vi "autofocus-mainvi.vi"() -> ()   [LabVIEW 2014]
uses:
  Stage Control/Stage SubVis/move stage.ctl
  autofocus-globals.vi
  tirf-lock-globals.vi
  <vilib>/Analysis/polynomials.llb/1D Polynomial Evaluation (DBL).vi
  <vilib>/Analysis/NI_AALPro.lvlib
panel:
  in  "Close laser shutter when autofocus is done?":bool
  in  "Close camera shutter during autofocus?":bool
  out "delta Z":dbl format="%#_13g"
  out "Calibration curve and fit":cluster{"QPD position":dbl[], "z (um)":ext[]}[](graph)
  out "Power":dbl format="%#_13g"
  out "Error Out":errorcluster
  in  "Error In":errorcluster
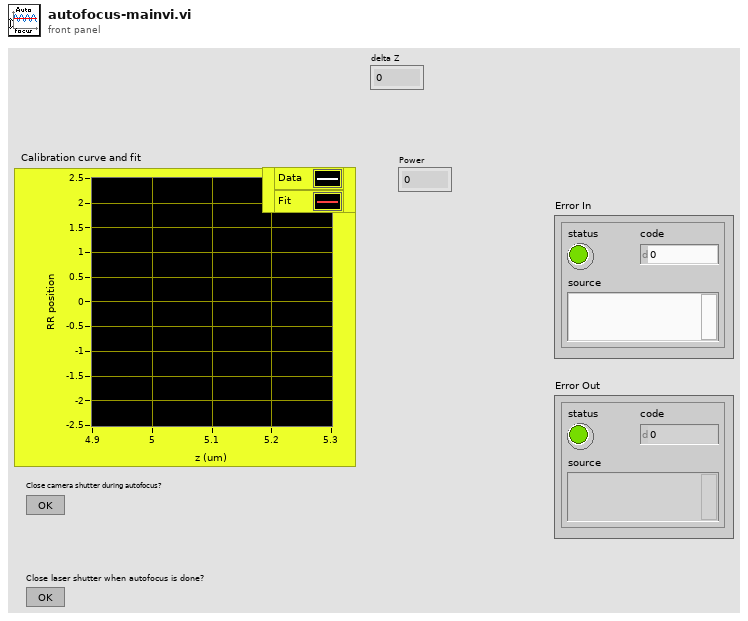
[diagram p1: front panel]
types:
  T1 = typedef "move stage.ctl" = cluster{"dx (um) (0 -> ignore)":ext, "dy (um) (0 -> ignore)":ext, "dz (um) (0 -> ignore)":ext, "Re-center x,y":bool, "Re-center z":bool, "x (um) (-1 -> ignore)":dbl, "y (um) (-1 -> ignore)":dbl, "z (um) (-1 -> ignore)":dbl}
  T2 = cluster{"QPD position":dbl[], "Best Polynomial Fit":dbl[]}
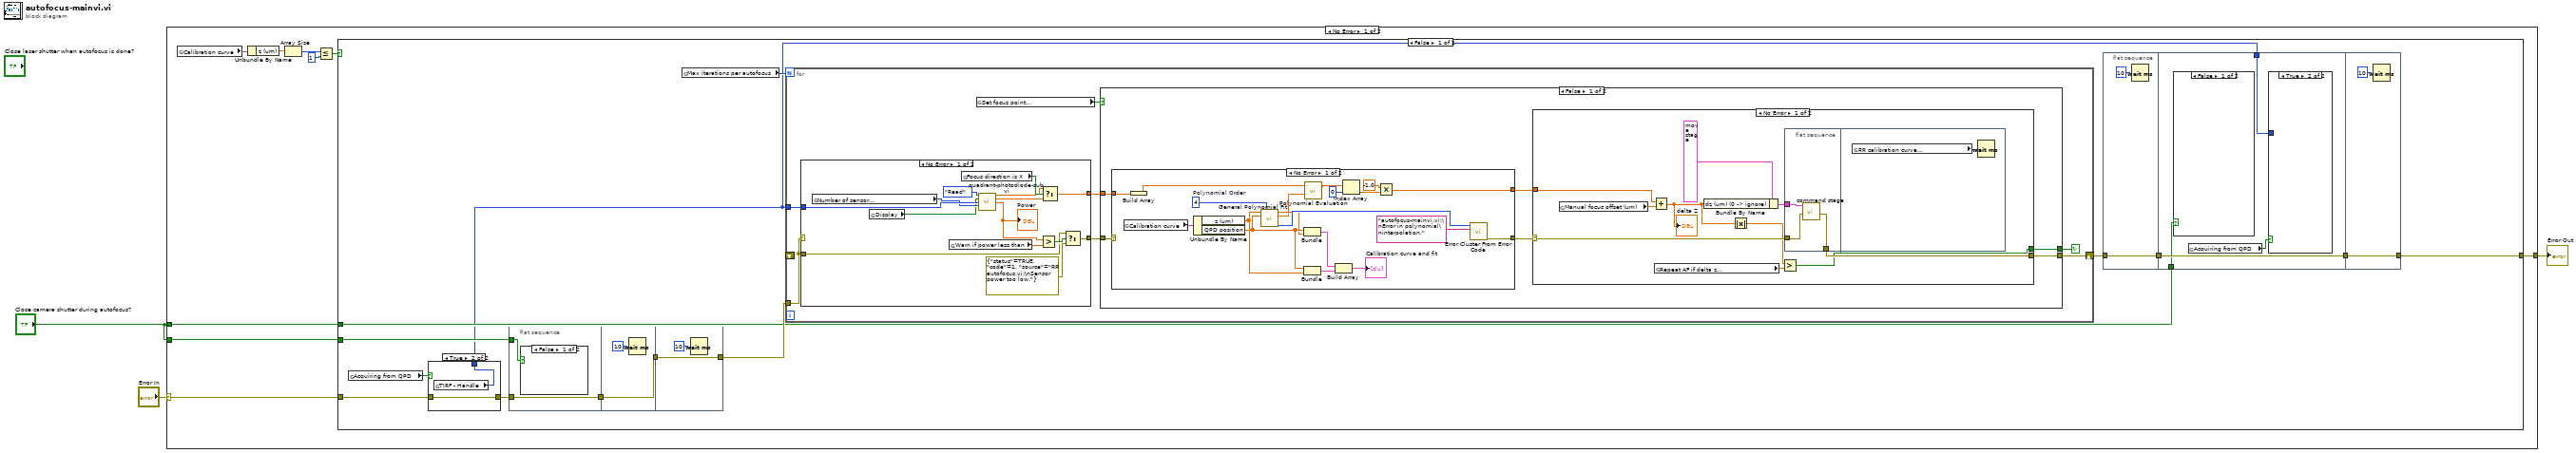
[diagram p0: block diagram]
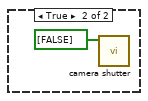
[diagram p2: hidden frame]
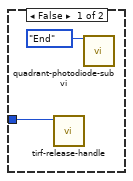
[diagram p3: hidden frame]
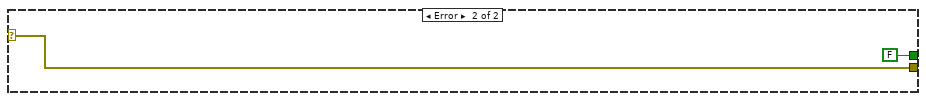
[diagram p4: hidden frame]
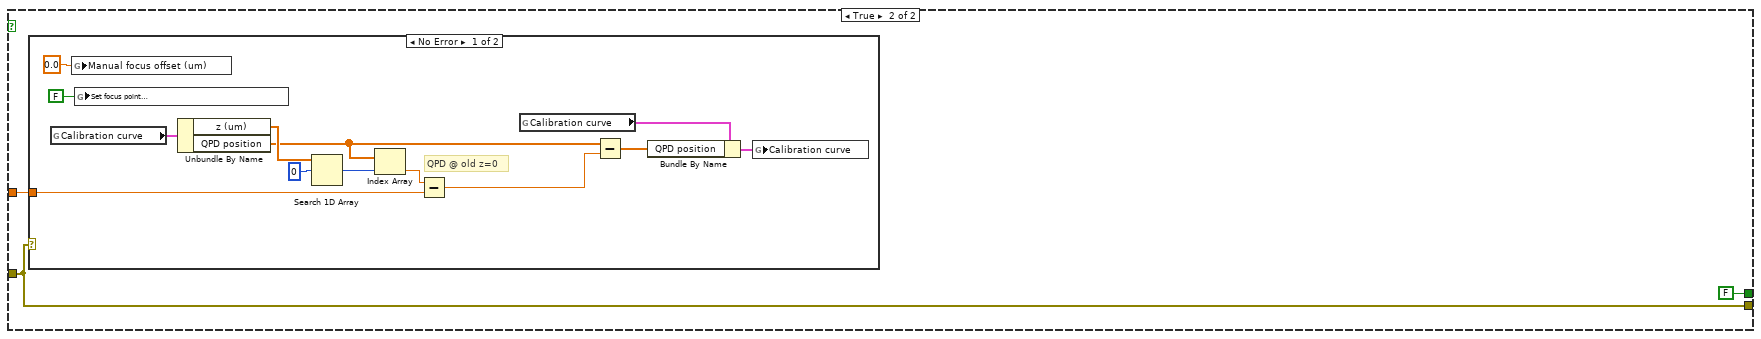
[diagram p6: hidden frame]
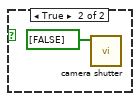
[diagram p9: hidden frame]
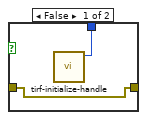
[diagram p10: hidden frame]
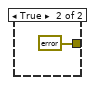
[diagram p11: hidden frame]
diagram:
  n1 = case shown="No Error" "Error In" {
    selector: "Error In" -> [w7 w131]
    tunnel: [w6 w131] -> w2
    tunnel: "Close camera shutter during autofocus?" -> [w5 _]
    tunnel: "Close camera shutter during autofocus?" -> [w4 _]
    frame No Error {
      n2 = global read "autofocus-globals.vi" "Calibration curve"() -> (w12:cluster{"z (um)":ext[], "QPD position":dbl[]})
      n3 = Unbundle By Name(w12) -> ("z (um)"=w9:ext[])
      n4 = Array Size(array=w9) -> (size(s)=w8:i32)
      n5 = Less Or Equal?(x=w8, y=1) -> (x <= y?=w10:bool)
      n6 = case shown="False" w10 {
        tunnel: w7 -> [w26 _]
        tunnel: [w17 errorcluster {"status"=TRUE, "code"=1, "source"="RR autofocus.vi:\nCan't autofocus because no\nautofocus calibration curve has been stored."} ("f")] -> w6
        tunnel: w5 -> [w16 _]
        tunnel: w4 -> [w15 _]
        frame False {
          n7 = global read "autofocus-globals.vi" "Acquiring from QPD"() -> (w25:bool)
          n8 = case shown="True" w25 {
            tunnel: w26 -> [w127 w129]
            tunnel: [w127 w129] -> w24
            tunnel: [w126 w128] -> w14
            frame False {
              n9 = call "tirf-initialize-handle.vi"() -> ("handle"=w126:i32)  [unwired: 11 in]
            }
            frame True {
              n10 = global read "autofocus-globals.vi" "TIRF - Handle"() -> (w128:u32)
            }
          }
          n11 = flat-sequence {
            tunnel: [w120] -> w23
            tunnel: w16 -> [w119]
            tunnel: w24 -> [w120]
            tunnel: w23 -> [w122]
            tunnel: [w122] -> w13
            tunnel: [w124] -> w21
            tunnel: w13 -> [w124]
            frame #0 {
              n12 = case shown="False" w119 {
                frame False {
                }
                frame True {
                  n13 = call "camera shutter.vi"("Array"=bool[] [FALSE]) -> ()  [unwired: 10 in, 1 out]
                }
              }
            }
            frame #1 {
              n14 = Wait (ms)(milliseconds to wait=u32 10) -> ()  [unwired: 1 out]
            }
            frame #2 {
              n15 = Wait (ms)(milliseconds to wait=u32 10) -> ()  [unwired: 1 out]
            }
          }
          n16 = global read "autofocus-globals.vi" "Max iterations per autofocus"() -> (w22:i32)
          n17 = for {
            N: w22 -> [_]
            tunnel: w21 -> [w38]
            shift-right: [w40] -> w20
            shift-left: _ -> [_]
            tunnel: w14 -> [w39]
            stop <- w41 continue-if-true
            n18 = case shown="No Error" w38 {
              selector: w38 -> [_ w118]
              tunnel: [w109 w118] -> w44
              tunnel: [w108 _] -> w42
              tunnel: w39 -> [w107 _]
              tunnel: w38 -> [w104 _]
              frame No Error {
                n19 = global read "autofocus-globals.vi" "Number of sensor\nreadings to average"() -> (w106:i32)
                n20 = global read "tirf-lock-globals.vi" "Display"() -> (w105:bool)
                n21 = global read "autofocus-globals.vi" "Warn if power less than"() -> (w111:dbl)
                n22 = global read "autofocus-globals.vi" "Focus direction is X"() -> (w116:bool)
                n23 = call "quadrant-photodiode-subvi.vi"("Mode"=enum16{"Start", "Read", "End"}."Read", "Display"=w105, "Handle"=w107, "Averages"=w106) -> ("coerced(x)"=w114:dbl, "coerced(y)"=w115:dbl, "Power (mw)"=w110:dbl)  [unwired: 9 in]
                "Power" <- w110
                n24 = Greater?(x=w110, y=w111) -> (0:w112:bool)
                n25 = Select(t=w114, s=w116, f=w115) -> (s? t:f=w108:dbl)
                n26 = Select(t=w104, s=w112, f=errorcluster {"status"=TRUE, "code"=1, "source"="RR autofocus.vi:\nSensor power too low."}) -> (s? t:f=w109:errorcluster)
              }
              frame Error {
              }
            }
            n27 = global read "autofocus-globals.vi" "Set focus point\nto current z position"() -> (w43:bool)
            n28 = case shown="False" w43 {
              tunnel: w44 -> [w50 w88]
              tunnel: w42 -> [w48 w89]
              tunnel: [w46 FALSE] -> w41
              tunnel: [w45 w88] -> w40
              frame False {
                n29 = case shown="No Error" w50 {
                  selector: w50 -> [_ w87]
                  tunnel: [w80 w87] -> w49
                  tunnel: w48 -> [w85 w86]
                  tunnel: [w76 w86] -> w47
                  frame No Error {
                    w83 = 4  # Polynomial Order
                    n30 = global read "autofocus-globals.vi" "Calibration curve"() -> (w84:cluster{"z (um)":ext[], "QPD position":dbl[]})
                    n31 = Build Array(w85) -> (w68:dbl[])
                    n32 = Unbundle By Name(w84) -> ("z (um)"=w75:ext[], "QPD position"=w74:dbl[])
                    n33 = call <vilib>:"General Polynomial Fit.vi"("Y"=w75, "polynomial order"=w83, "X"=w74) -> ("Best Polynomial Fit"=w73:dbl[], "Polynomial Coefficients"=w69:dbl[], "error"=w81:i32)  [unwired: 9 in, 1 out]
                    n34 = Bundle("QPD position"=w74, "Best Polynomial Fit"=w73) -> (w72:T2)  [unwired: 1 in]
                    n35 = Bundle("QPD position"=w74, "z (um)"=w75) -> (w71:cluster{"QPD position":dbl[], "z (um)":ext[]})  [unwired: 1 in]
                    n36 = call-poly <vilib>:"Polynomial Evaluation.vi"("P(x)"=w69, "A"=w68) -> ("P(A)"=w67:dbl[])  [unwired: 1 out]
                    n37 = Build Array(w72, w71) -> (→"Calibration curve and fit":cluster{"QPD position":dbl[], "z (um)":ext[]}[])
                    n38 = Index Array(array=w67, index=0) -> (element=w78:dbl)
                    n39 = Multiply(x=-1.0, y=w78) -> (x*y=w76:dbl)
                    n40 = call <vilib>:"Error Cluster From Error Code.vi"("error message (\"\")"="autofocus-mainvi.vi:\nError in polynomial\ninterpolation." ("error message (\"\")"), "error code (0)"=w81) -> ("error out"=w80:errorcluster)  [unwired: 2 in, 5 out]
                  }
                  frame Error {
                  }
                }
                n41 = case shown="No Error" w49 {
                  selector: w49 -> [w60 w66]
                  tunnel: [w59 w66] -> w45
                  tunnel: w47 -> [w57 _]
                  tunnel: [w51 FALSE] -> w46
                  frame No Error {
                    n42 = global read "autofocus-globals.vi" "Manual focus offset (um)"() -> (w58:dbl)
                    n43 = Add(x=w57, y=w58) -> (x+y=w54:dbl)
                    "delta Z" <- w54
                    n44 = global read "autofocus-globals.vi" "Repeat AF if delta z \ngreater than (um)"() -> (w52:dbl)
                    n45 = Bundle By Name(cluster=T1 {"dx (um) (0 -> ignore)"=0.0, "dy (um) (0 -> ignore)"=0.0, "dz (um) (0 -> ignore)"=0.0, "Re-center x,y"=FALSE, "Re-center z"=FALSE, "x (um) (-1 -> ignore)"=-1.0, "y (um) (-1 -> ignore)"=-1.0, "z (um) (-1 -> ignore)"=-1.0} ("Command Stage"), "dz (um) (0 -> ignore)"=w54) -> (w55:T1)
                    n46 = Absolute Value(x=w54) -> (abs(x)=w53:dbl)
                    n47 = Greater?(x=w53, y=w52) -> (0:w51:bool)
                    n48 = flat-sequence {
                      tunnel: w60 -> [w63]
                      tunnel: [w62] -> w59
                      tunnel: w55 -> [w61]
                      frame #0 {
                        n49 = call "command stage.vi"("Error In"=w63, "Command Stage"=w61) -> ("Error Out"=w62:errorcluster)  [unwired: 9 in]
                      }
                      frame #1 {
                        n50 = global read "autofocus-globals.vi" "RR calibration curve\nsettle time (ms)"() -> (w64:u16)
                        n51 = Wait (ms)(milliseconds to wait=w64) -> ()  [unwired: 1 out]
                      }
                    }
                  }
                  frame Error {
                  }
                }
              }
              frame True {
                n52 = case shown="No Error" w88 {
                  tunnel: w89 -> [w96 _]
                  frame No Error {
                    # "QPD @ old z=0"
                    n53 = global read "autofocus-globals.vi" "Calibration curve"() -> (w103:cluster{"z (um)":ext[], "QPD position":dbl[]})
                    n54 = global write "autofocus-globals.vi" "Manual focus offset (um)"(0.0) -> ()
                    n55 = global write "autofocus-globals.vi" "Set focus point\nto current z position"(FALSE) -> ()
                    n56 = Unbundle By Name(w103) -> ("z (um)"=w101:ext[], "QPD position"=w97:dbl[])
                    n57 = Search 1D Array(1D array=w101, element=0) -> (index of element=w102:i32)  [unwired: 1 in]
                    n58 = Index Array(array=w97, index=w102) -> (element=w99:dbl)
                    n59 = Subtract(x=w99, y=w96) -> (x-y=w98:dbl)
                    n60 = global read "autofocus-globals.vi" "Calibration curve"() -> (w95:cluster{"z (um)":ext[], "QPD position":dbl[]})
                    n61 = Subtract(x=w97, y=w98) -> (x-y=w94:dbl[])
                    n62 = Bundle By Name(cluster=w95, "QPD position"=w94) -> (w93:cluster{"z (um)":ext[], "QPD position":dbl[]})
                    n63 = global write "autofocus-globals.vi" "Calibration curve"(w93) -> ()
                  }
                  frame Error {
                  }
                }
              }
            }
          }
          n64 = flat-sequence {
            tunnel: [w28] -> w18
            tunnel: w20 -> [w28]
            tunnel: [w32] -> w19
            tunnel: w18 -> [w32]
            tunnel: w15 -> [w30]
            tunnel: w14 -> [w29]
            tunnel: w19 -> [w37]
            tunnel: [w37] -> w17
            frame #0 {
              n65 = Wait (ms)(milliseconds to wait=u32 10) -> ()  [unwired: 1 out]
            }
            frame #1 {
              n66 = case shown="False" w30 {
                frame False {
                }
                frame True {
                  n67 = call "camera shutter.vi"("Array"=bool[] [FALSE]) -> ()  [unwired: 10 in, 1 out]
                }
              }
              n68 = global read "autofocus-globals.vi" "Acquiring from QPD"() -> (w31:bool)
              n69 = case shown="True" w31 {
                tunnel: w29 -> [w34 _]
                frame False {
                  n70 = call "tirf-release-handle.vi"("handle"=w34) -> ()  [unwired: 11 in]
                  n71 = call "quadrant-photodiode-subvi.vi"("Mode"=enum16{"Start", "Read", "End"}."End") -> ()  [unwired: 12 in, 3 out]
                }
                frame True {
                }
              }
            }
            frame #2 {
              n72 = Wait (ms)(milliseconds to wait=u32 10) -> ()  [unwired: 1 out]
            }
          }
        }
        frame True {
        }
      }
    }
    frame Error {
    }
  }
  "Error Out" <- w2
